vi "TagMetadataToImage.vi"(8 "error in (no error)":errorcluster, 10 "Image In":T1, 11 "DemoStage in":refnum<class "DemoStage.lvclass">) -> (0 "error out":errorcluster, 2 "Image Out":T1, 3 "DemoStage out":refnum<class "DemoStage.lvclass">)   [LabVIEW 2020, in "DemoStage.lvlib" / "DemoStage.lvclass"]
uses:
  DemoStage.lvclass
  <vilib>/vision/Image Controls.llb/IMAQ Image.ctl
  DemoStage.lvclass/DemoStage.ctl
  Hardware Abstraction Layer/Component/Stage/Stage/Stage.lvclass
panel:
  out "Custom Data Out":string
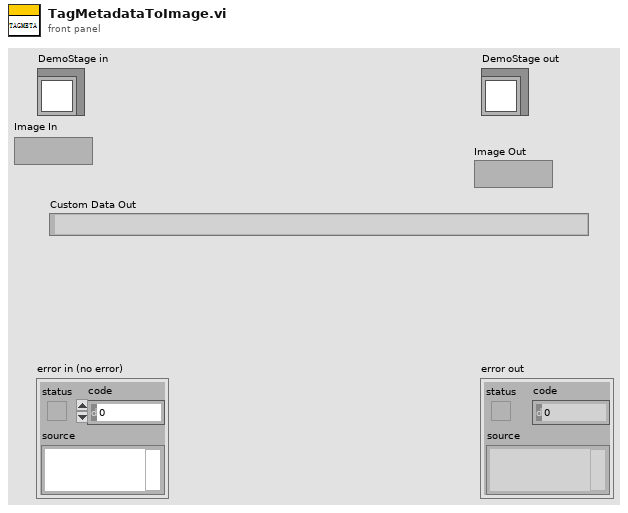
[diagram p1: front panel]
types:
  T1 = typedef "IMAQ Image.ctl" = refnum<image>
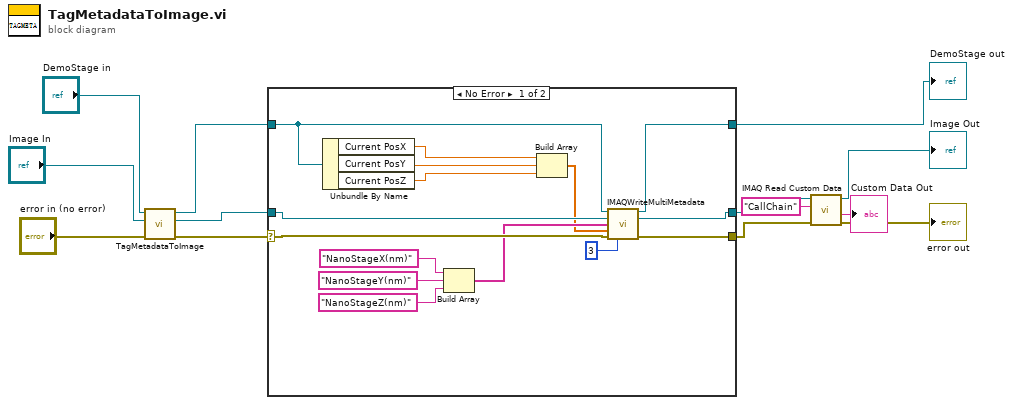
[diagram p0: block diagram]
diagram:
  n1 = call-parent "TagMetadataToImage.vi"("error in (no error)"="error in (no error)", "Image In"="Image In", "Device in"="DemoStage in") -> ("error out"=w10:errorcluster, "Image Out"=w9:T1, "Device out"=w8:refnum<class "DemoStage.lvclass">)  [unwired: 6 in]
  n2 = case shown="No Error" w10 {
    selector: w10 -> [w28 w31]
    tunnel: [w26 w31] -> w6
    tunnel: w9 -> [w27 w29]
    tunnel: [w25 w30] -> w7
    tunnel: w8 -> [w15 w30]
    tunnel: [w24 w29] -> w4
    frame No Error {
      n3 = Unbundle By Name(w15) -> ("Current PosX"=w18:dbl, "Current PosY"=w17:dbl, "Current PosZ"=w16:dbl)
      n4 = Build Array("NanoStageX(nm)" ("Key"), "NanoStageY(nm)" ("Key"), "NanoStageZ(nm)" ("Key")) -> (w19:string[])
      n5 = Build Array(w18, w17, w16) -> (w14:dbl[])
      n6 = call-dynamic "IMAQWriteMultiMetadata.vi"("GRMActor in"=w15, "Image In"=w27, "Keys"=w19, "Values"=w14, "error in (no error)"=w28, "precision (6)"=i16 3) -> ("GRMActor out"=w25:refnum<class "DemoStage.lvclass">, "Image Out"=w24:T1, "error out"=w26:errorcluster)  [unwired: 7 in]
    }
    frame Error {
    }
  }
  "DemoStage out" <- w7
  n7 = call "IMAQ Read Custom Data"("error in (no error)"=w6, "Key"="CallChain", "Image"=w4) -> ("error out"=→"error out":errorcluster, "Custom Data Out"=→"Custom Data Out":string, "Image (duplicate)"=→"Image Out":T1)  [unwired: 6 in]
